vi "Tokenize.vi"(10 "Policy":T3=enum."lenient", 11 "Input":string="https://cdn-*.example.com/*.jpg") -> (0 "error out":errorcluster, 3 "Token List":T1[](array[typedef]))   [LabVIEW 2020, in "Stream.lvlib" / "URLPattern.lvclass"]
uses:
  URLPattern.lvclass
  Tokenize Policy.ctl
  Token.ctl
  Token Type.ctl
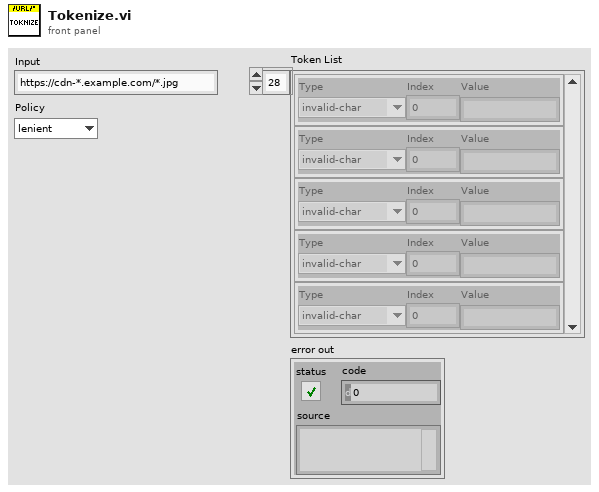
[diagram p1: front panel]
types:
  T1 = typedef "Stream.lvlib/URLPattern.lvclass/Token.ctl" = cluster{"Type":T2, "Index":i32, "Value":string}
  T2 = typedef "Stream.lvlib/URLPattern.lvclass/Token Type.ctl" = enum16{"invalid-char", "open", "close", "regexp", "name", "char", "escaped-char", "other-modifier", "asterisk", "end"}
  T3 = typedef "Stream.lvlib/URLPattern.lvclass/Tokenize Policy.ctl" = enum16{"strict", "lenient"}
  T4 = typedef "Stream.lvlib/URLPattern.lvclass/Tokenizer.ctl" = cluster{"Input":string, "Policy":T3, "Token List":refnum<queue>, "Index":i32, "Next Index":i32, "Code Point":u32, "Length":i32}
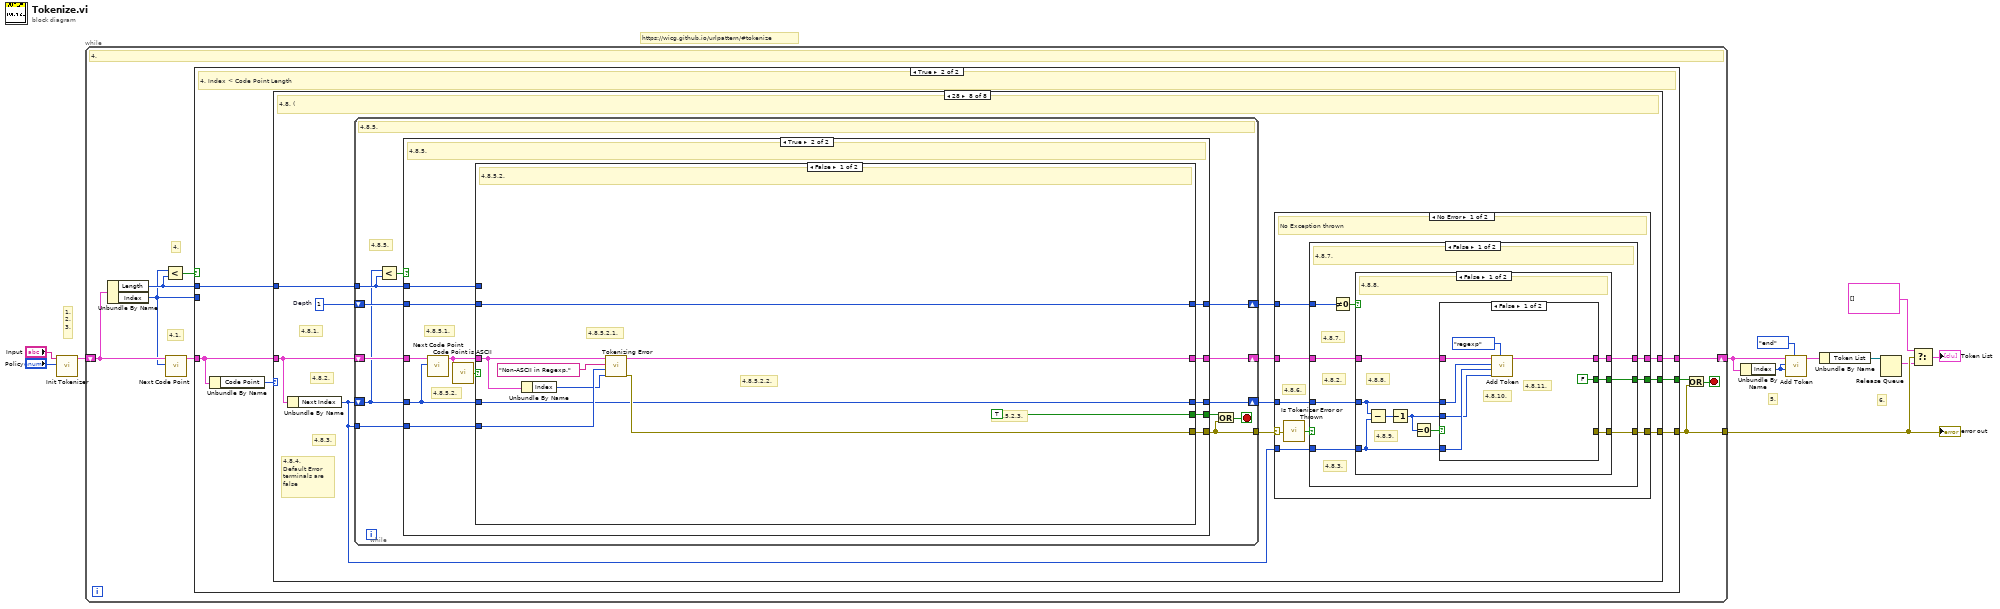
[diagram p0: block diagram]
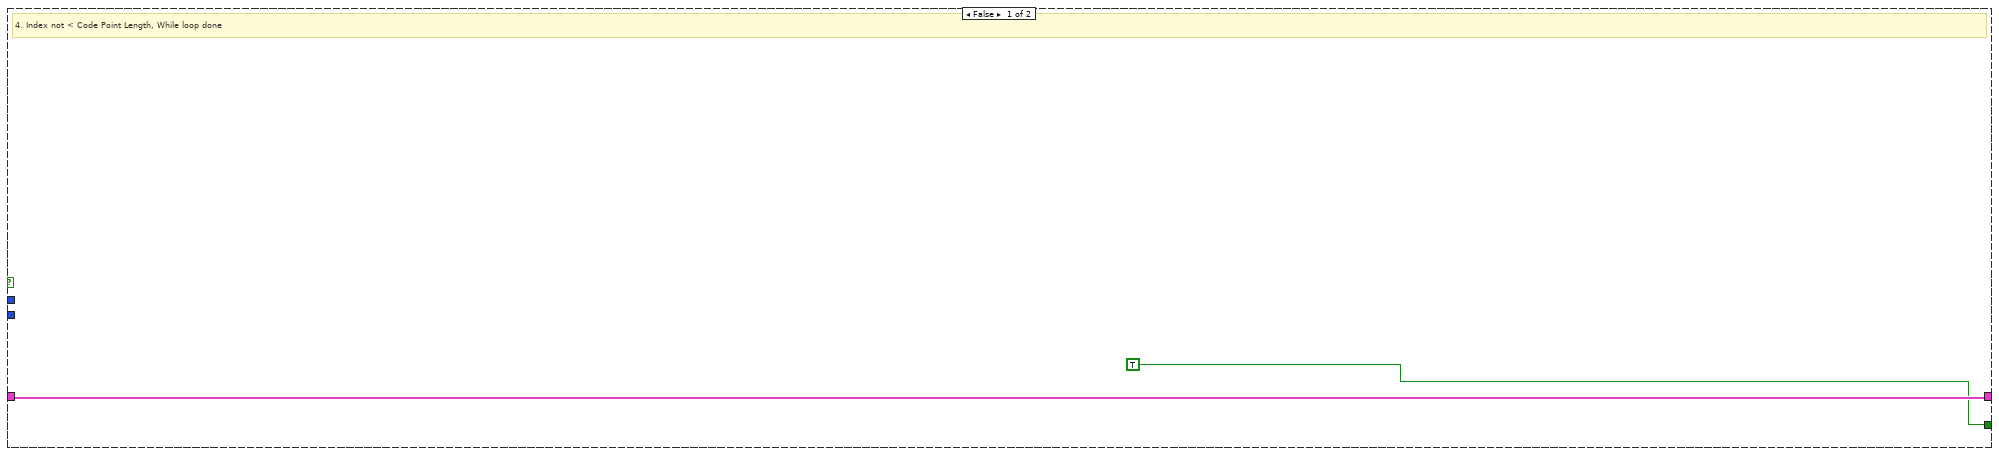
[diagram p2: hidden frame]
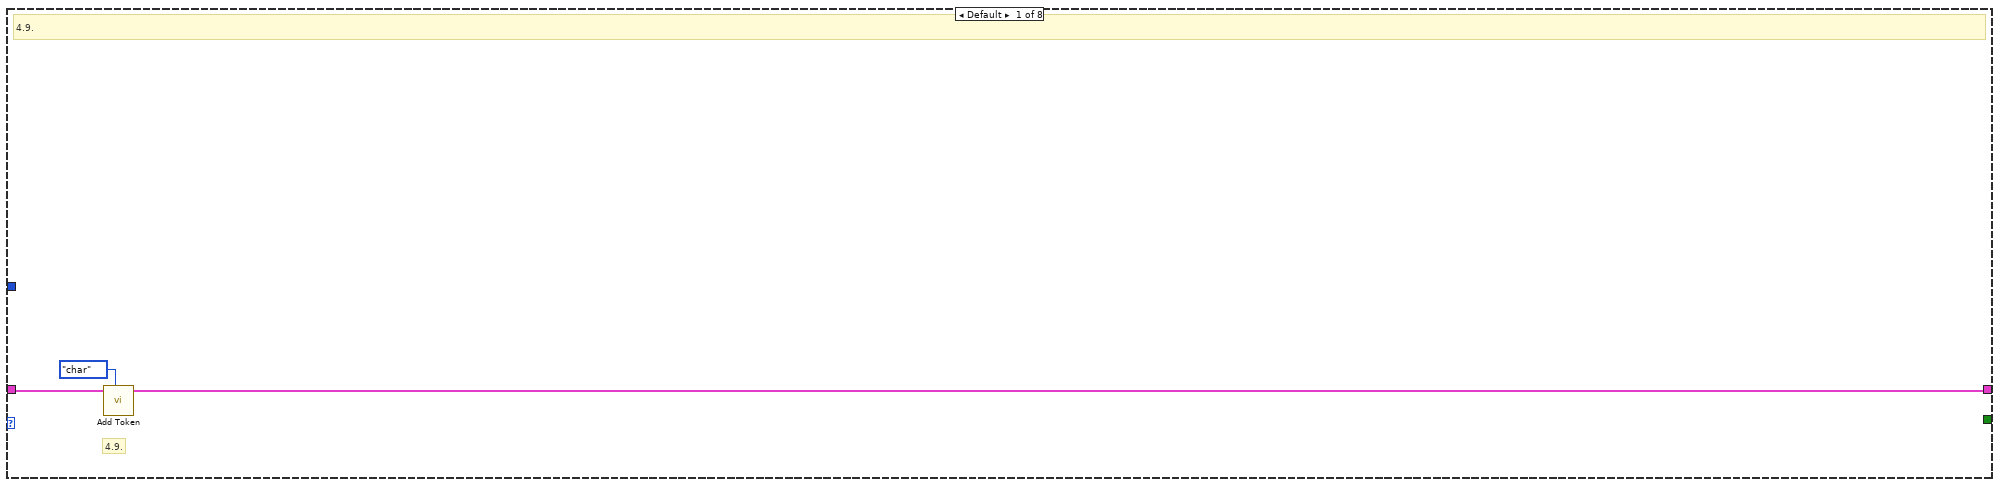
[diagram p3: hidden frame]
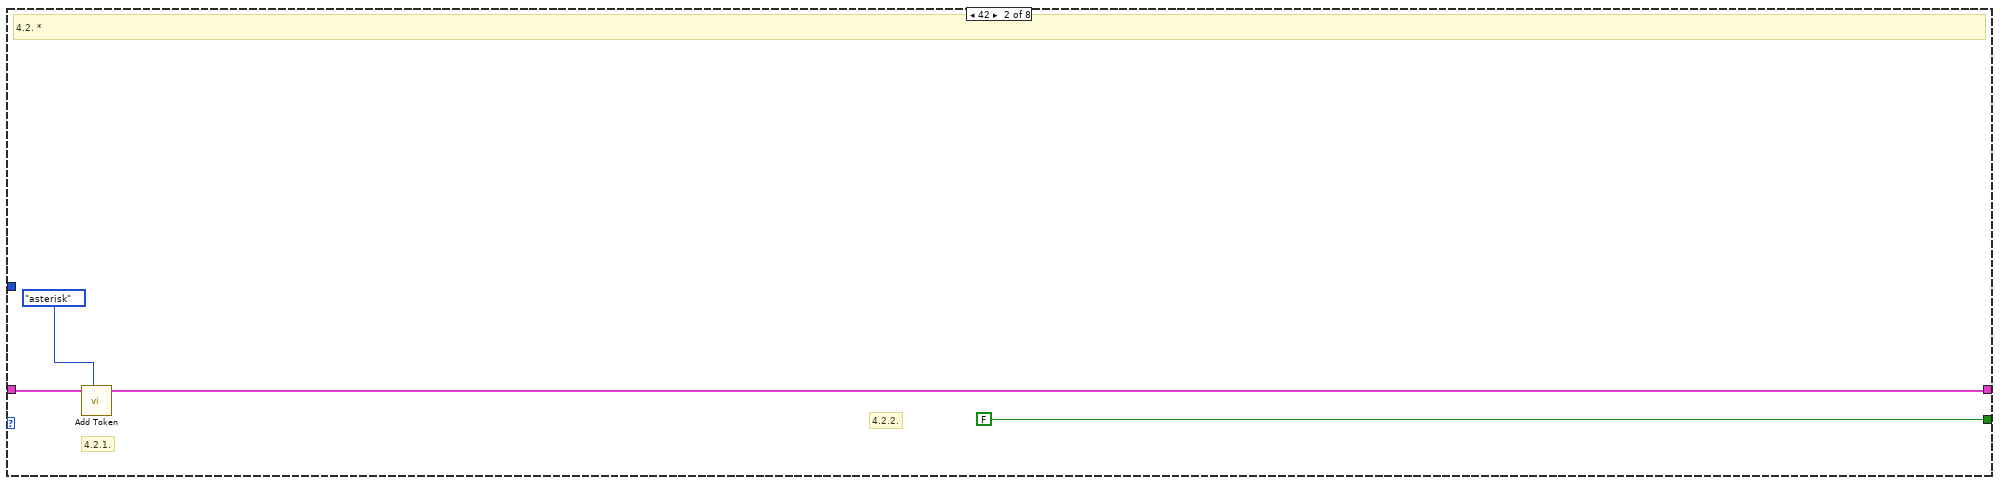
[diagram p4: hidden frame]
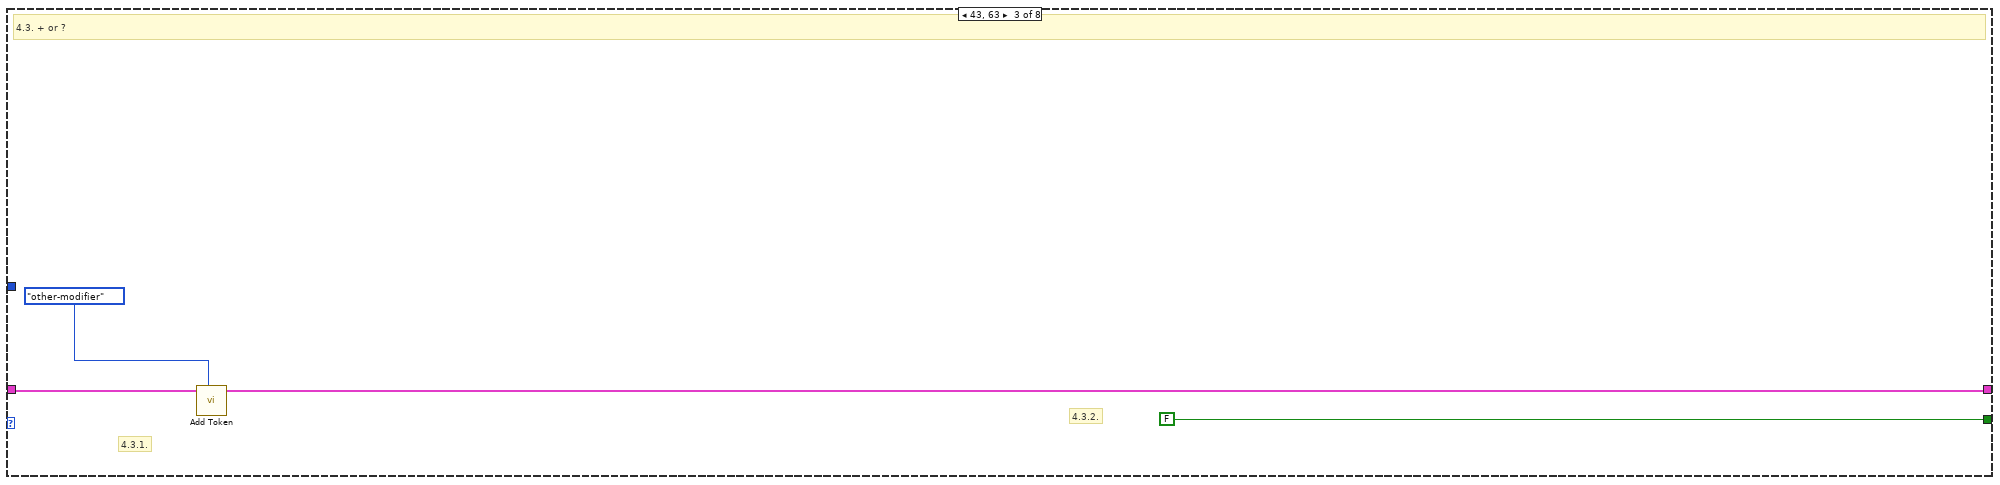
[diagram p5: hidden frame]
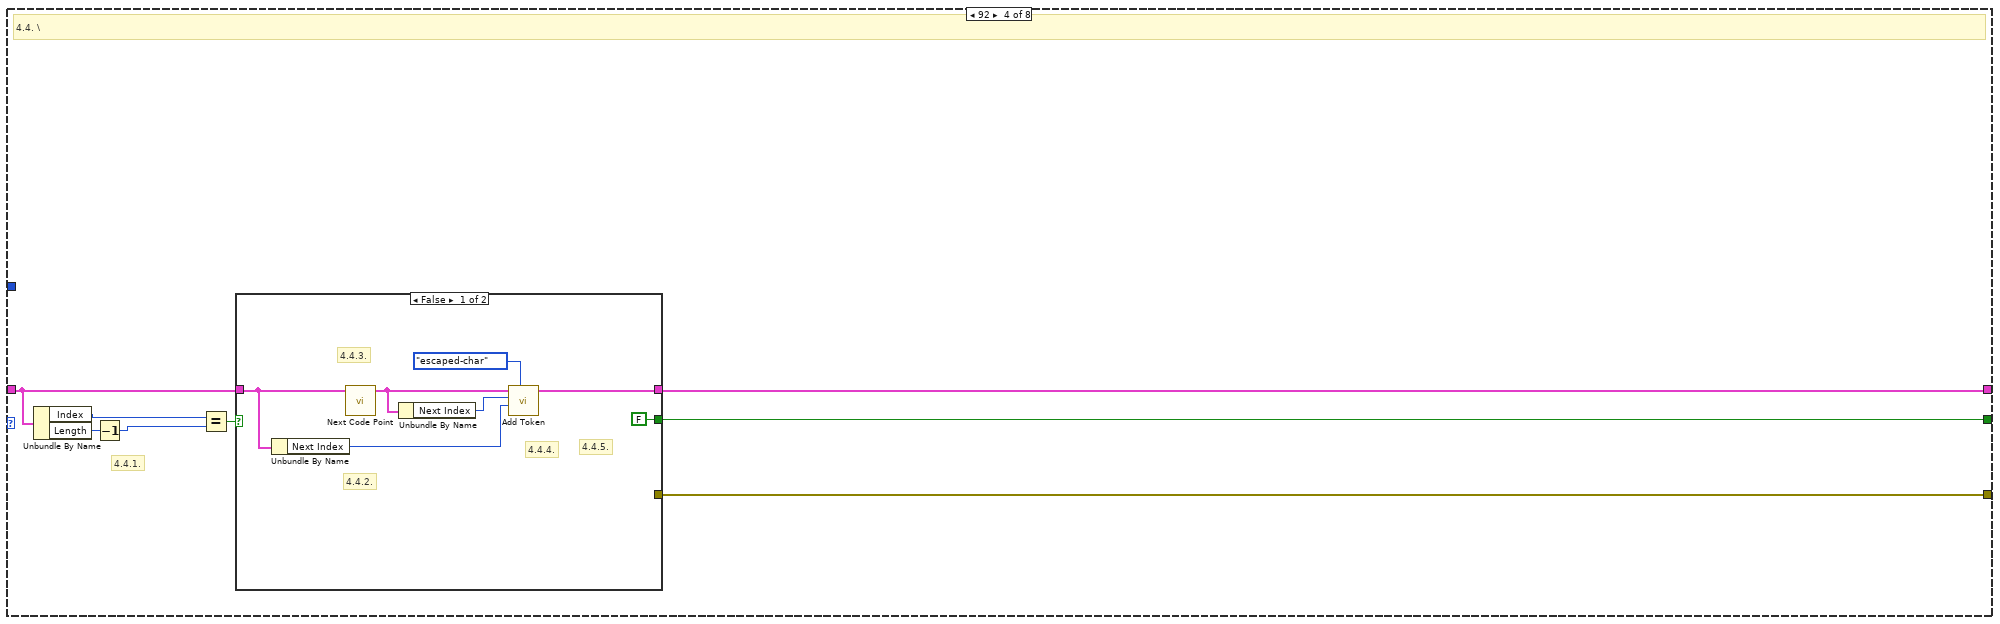
[diagram p6: hidden frame]
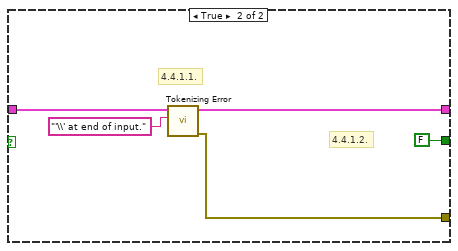
[diagram p7: hidden frame]
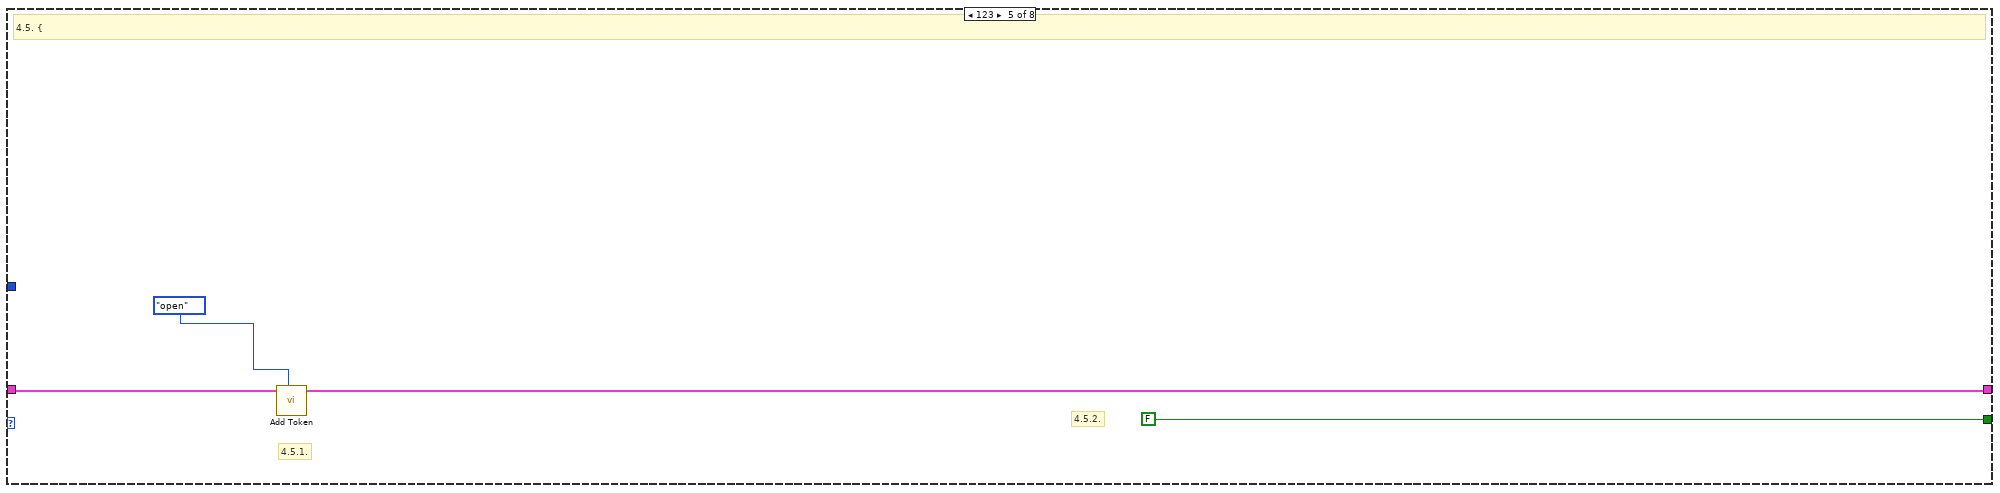
[diagram p8: hidden frame]
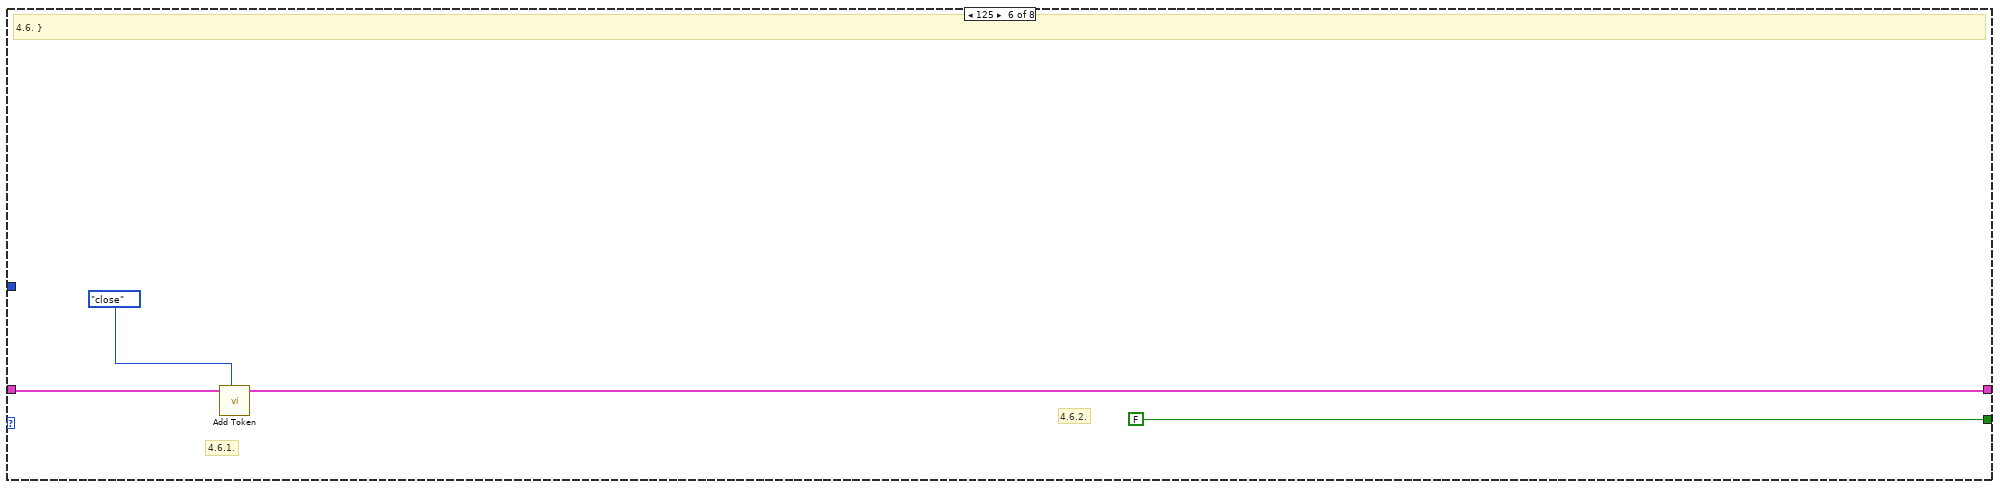
[diagram p9: hidden frame]
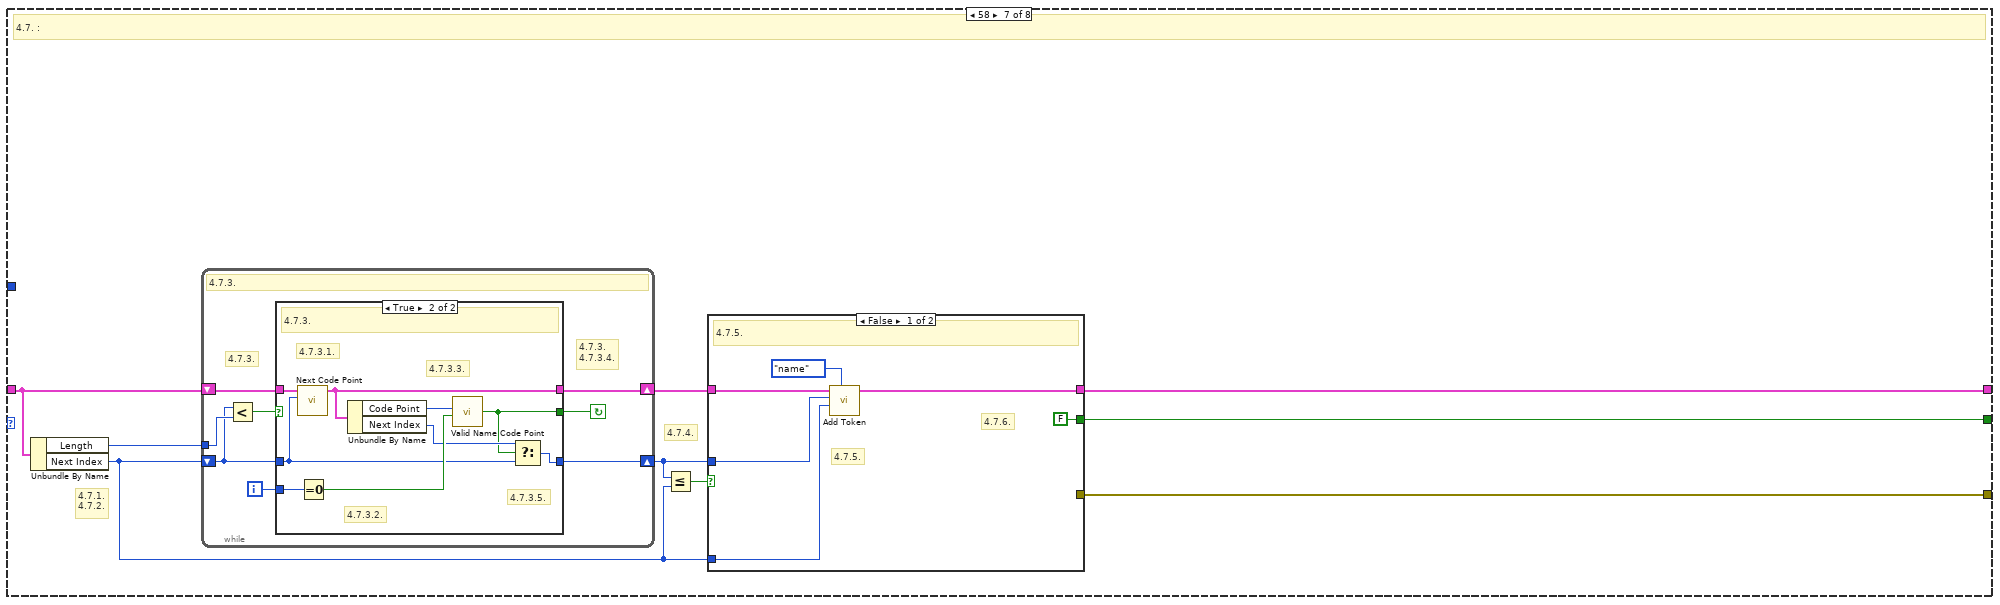
[diagram p10: hidden frame]
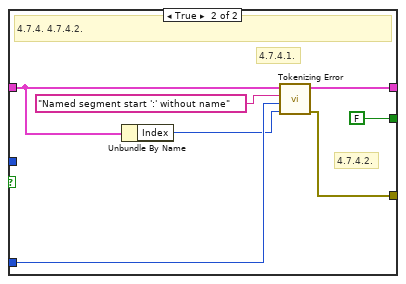
[diagram p11: hidden frame]
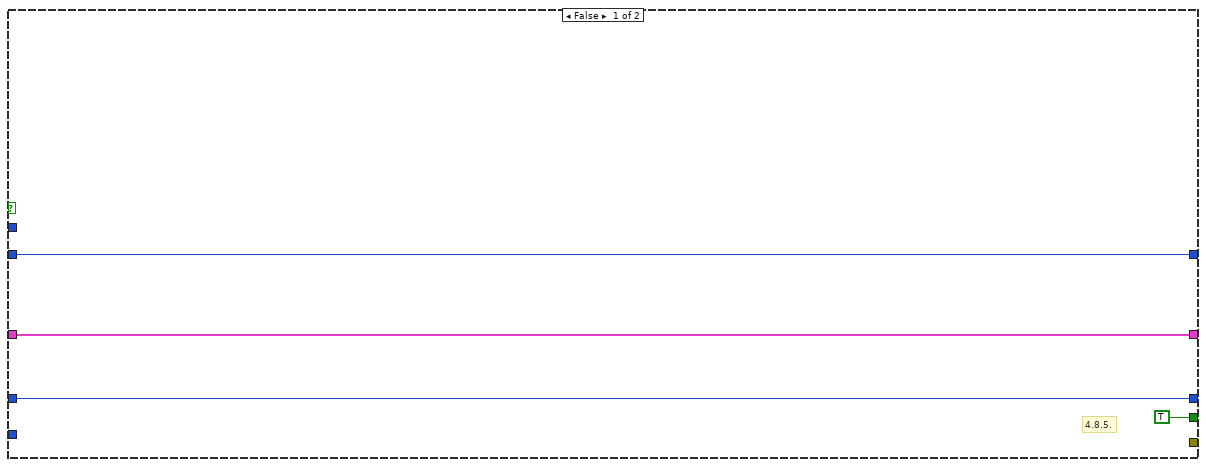
[diagram p13: hidden frame]
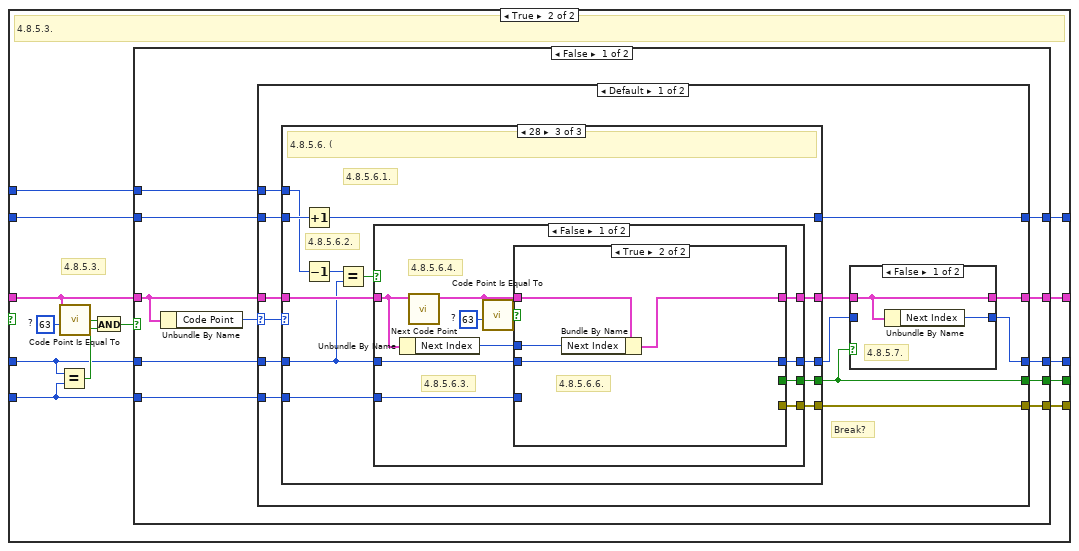
[diagram p14: hidden frame]
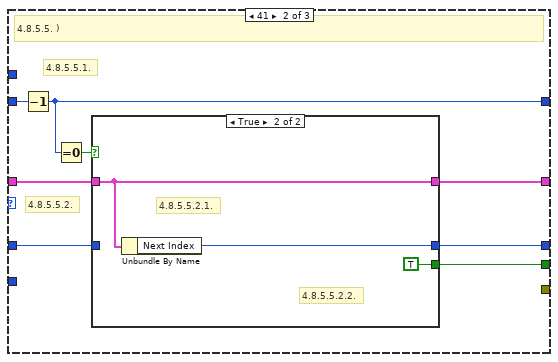
[diagram p17: hidden frame]
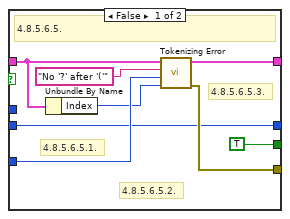
[diagram p19: hidden frame]
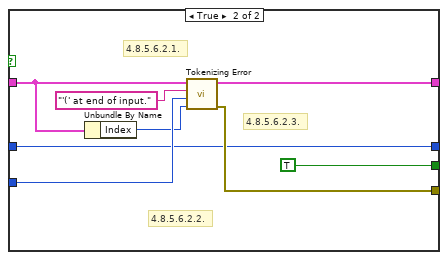
[diagram p20: hidden frame]
diagram:
  # "6."
  # "5."
  # "https://wicg.github.io/urlpattern/#tokenize"
  # "1.\n2.\n3."
  n1 = call "Init Tokenizer.vi"("Policy"="Policy", "Input"="Input") -> ("Tokenizer"=w9:T4)  [unwired: 9 in]
  n2 = while {
    shift-right: [w20] -> w2
    shift-left: w9 -> [w16]
    tunnel: [w17] -> w12
    stop <- w18 stop-if-true
    # "4.1."
    # "4."
    # "4."
    n3 = Unbundle By Name(w16) -> ("Length"=w14:i32, "Index"=w13:i32)
    n4 = Less?(x=w13, y=w14) -> (x < y?=w21:bool)
    n5 = call "Next Code Point.vi"("Index"=w13, "Tokenizer In"=w16) -> ("Tokenizer"=w15:T4)  [unwired: 9 in]
    n6 = case shown="True" w21 {
      tunnel: w13 -> [_ _]
      tunnel: w15 -> [w23 w28]
      tunnel: [w23 w27] -> w20
      tunnel: [TRUE w24] -> w19
      tunnel: [_ w26] -> w17
      tunnel: w14 -> [_ w25]
      frame False {
        # "4. Index not < Code Point Length, While loop done"
      }
      frame True {
        # "4. Index < Code Point Length"
        n7 = Unbundle By Name(w28) -> ("Code Point"=w29:u32)
        n8 = case shown="28" w29 {
          tunnel: w28 -> [w32 w36 w40 w45 w64 w68 w77 w120]
          tunnel: [w30 w34 w38 w42 w62 w66 w73 w114] -> w27
          tunnel: [_ _ _ w43 _ _ w72 w116] -> w26
          tunnel: w25 -> [_ _ _ _ _ _ _ w119]
          tunnel: [_ FALSE FALSE w41 FALSE FALSE w69 w117] -> w24
          frame Default {
            # "4.9."
            # "4.9."
            n9 = call "Add Token.vi"("Token Type"=Token_Type."char", "Tokenizer In"=w32) -> ("Tokenizer"=w30:T4)  [unwired: 9 in]
          }
          frame 42 {
            # "4.2.2."
            # "4.2.1."
            # "4.2. *"
            n10 = call "Add Token.vi"("Token Type"=Token_Type."asterisk", "Tokenizer In"=w36) -> ("Tokenizer"=w34:T4)  [unwired: 9 in]
          }
          frame 43, 63 {
            # "4.3.2."
            # "4.3.1."
            # "4.3. + or ?"
            n11 = call "Add Token.vi"("Token Type"=Token_Type."other-modifier", "Tokenizer In"=w40) -> ("Tokenizer"=w38:T4)  [unwired: 9 in]
          }
          frame 92 {
            # "4.4.1."
            # "4.4. \\"
            n12 = Unbundle By Name(w45) -> ("Index"=w46:i32, "Length"=w48:i32)
            n13 = Decrement(x=w48) -> (x-1=w47:i32)
            n14 = Equal?(x=w46, y=w47) -> (x = y?=w44:bool)
            n15 = case shown="False" w44 {
              tunnel: w45 -> [w55 w60]
              tunnel: [_ w57] -> w43
              tunnel: [w53 w58] -> w42
              tunnel: [FALSE FALSE] -> w41
              frame False {
                # "4.4.5."
                # "4.4.4."
                # "4.4.3."
                # "4.4.2."
                n16 = Unbundle By Name(w55) -> ("Next Index"=w52:i32)
                n17 = call "Next Code Point.vi"("Tokenizer In"=w55) -> ("Tokenizer"=w51:T4)  [unwired: 10 in]
                n18 = Unbundle By Name(w51) -> ("Next Index"=w50:i32)
                n19 = call "Add Token.vi"("Token Type"=Token_Type."escaped-char", "Value Position"=w52, "Next Position"=w50, "Tokenizer In"=w51) -> ("Tokenizer"=w53:T4)  [unwired: 7 in]
              }
              frame True {
                # "4.4.1.2."
                # "4.4.1.1."
                n20 = call "Tokenizing Error.vi"("Reason"="'\\' at end of input.", "Tokenizer In"=w60) -> ("error out"=w57:errorcluster, "Tokenizer"=w58:T4)  [unwired: 8 in]
              }
            }
          }
          frame 123 {
            # "4.5.2."
            # "4.5.1."
            # "4.5. {"
            n21 = call "Add Token.vi"("Token Type"=Token_Type."open", "Tokenizer In"=w64) -> ("Tokenizer"=w62:T4)  [unwired: 9 in]
          }
          frame 125 {
            # "4.6.2."
            # "4.6.1."
            # "4.6. }"
            n22 = call "Add Token.vi"("Token Type"=Token_Type."close", "Tokenizer In"=w68) -> ("Tokenizer"=w66:T4)  [unwired: 9 in]
          }
          frame 58 {
            # "4.7.4."
            # "4.7.1.\n4.7.2."
            # "4.7. :"
            n23 = Unbundle By Name(w77) -> ("Length"=w76:i32, "Next Index"=w71:i32)
            n24 = while {
              shift-right: [w95] -> w70
              shift-left: w71 -> [w92]
              shift-right: [w94] -> w74
              shift-left: w77 -> [w98]
              tunnel: w76 -> [w93]
              i -> [w97]
              stop <- w96 continue-if-true
              # "4.7.3.\n4.7.3.4."
              # "4.7.3."
              # "4.7.3."
              n25 = Less?(x=w92, y=w93) -> (x < y?=w91:bool)
              n26 = case shown="True" w91 {
                selector: w91 -> [w101 _]
                tunnel: w98 -> [w100 w110]
                tunnel: w97 -> [_ w109]
                tunnel: [w101 w105] -> w96
                tunnel: [w99 w104] -> w95
                tunnel: [w100 w103] -> w94
                tunnel: w92 -> [w99 w102]
                frame False {
                  # "4.7.3."
                }
                frame True {
                  # "4.7.3.5."
                  # "4.7.3.3."
                  # "4.7.3.2."
                  # "4.7.3.1."
                  # "4.7.3."
                  n27 = call "Next Code Point.vi"("Index"=w102, "Tokenizer In"=w110) -> ("Tokenizer"=w103:T4)  [unwired: 9 in]
                  n28 = Equal To 0?(x=w109) -> (x = 0?=w107:bool)
                  n29 = Unbundle By Name(w103) -> ("Code Point"=w108:u32, "Next Index"=w106:i32)
                  n30 = call "Valid Name Code Point.vi"("First"=w107, "Code Point"=w108) -> ("Valid?"=w105:bool)  [unwired: 2 in]
                  n31 = Select(t=w106, s=w105, f=w102) -> (s? t:f=w104:i32)
                }
              }
            }
            n32 = Less Or Equal?(x=w70, y=w71) -> (x <= y?=w75:bool)
            n33 = case shown="False" w75 {
              tunnel: w74 -> [w80 w86]
              tunnel: [w83 w90] -> w73
              tunnel: [_ w89] -> w72
              tunnel: w71 -> [w78 w87]
              tunnel: w70 -> [w81 _]
              tunnel: [FALSE FALSE] -> w69
              frame False {
                # "4.7.6."
                # "4.7.5."
                # "4.7.5."
                n34 = call "Add Token.vi"("Token Type"=Token_Type."name", "Value Position"=w78, "Next Position"=w81, "Tokenizer In"=w80) -> ("Tokenizer"=w83:T4)  [unwired: 7 in]
              }
              frame True {
                # "4.7.4.2."
                # "4.7.4.1."
                # "4.7.4. 4.7.4.2."
                n35 = Unbundle By Name(w86) -> ("Index"=w85:i32)
                n36 = call "Tokenizing Error.vi"("Value Position"=w85, "Next Position"=w87, "Reason"="Named segment start ':' without name", "Tokenizer In"=w86) -> ("error out"=w89:errorcluster, "Tokenizer"=w90:T4)  [unwired: 6 in]
              }
            }
          }
          frame 40 {
            w121 = 1  # Depth
            # "4.8.3."
            # "4.8.4.\nDefault Error terminals are false"
            # "4.8.1."
            # "4.8.2."
            # "4.8. ("
            n37 = Unbundle By Name(w120) -> ("Next Index"=w111:i32)
            n38 = while {
              shift-right: [w129] -> w112
              shift-left: w121 -> [w132]
              shift-right: [w128] -> w113
              shift-left: w111 -> [w126]
              tunnel: w111 -> [w131]
              shift-right: [w130] -> w115
              shift-left: w120 -> [w133]
              tunnel: [w122] -> w118
              tunnel: w119 -> [w127]
              stop <- w123 stop-if-true
              # "4.8.5."
              # "4.8.5."
              n39 = Less?(x=w126, y=w127) -> (x < y?=w125:bool)
              n40 = case shown="True" w125 {
                tunnel: w133 -> [w136 w149]
                tunnel: w132 -> [w137 w146]
                tunnel: w131 -> [_ w145]
                tunnel: [w136 w144] -> w130
                tunnel: [w137 w143] -> w129
                tunnel: [w135 w142] -> w128
                tunnel: [TRUE w141] -> w124
                tunnel: [_ w140] -> w122
                tunnel: w127 -> [_ w139]
                tunnel: w126 -> [w135 w138]
                frame False {
                  # "4.8.5."
                }
                frame True {
                  # "4.8.5.2."
                  # "4.8.5.1."
                  # "4.8.5."
                  n41 = call "Next Code Point.vi"("Index"=w138, "Tokenizer In"=w149) -> ("Tokenizer"=w147:T4)  [unwired: 9 in]
                  n42 = call "Code Point is ASCII.vi"("Tokenizer"=w147) -> ("ASCII?"=w148:bool)
                  n43 = case shown="False" w148 {
                    tunnel: w147 -> [w156 w168]
                    tunnel: w146 -> [w152 w162]
                    tunnel: w145 -> [w157 w166]
                    tunnel: [w154 w164] -> w140
                    tunnel: [w153 w165] -> w144
                    tunnel: [w152 w161] -> w143
                    tunnel: w138 -> [w151 w167]
                    tunnel: [w151 w163] -> w142
                    tunnel: w139 -> [_ w160]
                    tunnel: [TRUE w159] -> w141
                    frame False {
                      # "4.8.5.2.3."
                      # "4.8.5.2.2."
                      # "4.8.5.2.1."
                      # "4.8.5.2."
                      n44 = Unbundle By Name(w156) -> ("Index"=w155:i32)
                      n45 = call "Tokenizing Error.vi"("Value Position"=w155, "Next Position"=w157, "Reason"="Non-ASCII in Regexp.", "Tokenizer In"=w156) -> ("error out"=w154:errorcluster, "Tokenizer"=w153:T4)  [unwired: 6 in]
                    }
                    frame True {
                      w172 = u32 63  # ?
                      # "4.8.5.3."
                      # "4.8.5.3."
                      n46 = Equal?(x=w167, y=w166) -> (x = y?=w170:bool)
                      n47 = call "Code Point Is Equal To.vi"("Code Point"=w172, "Tokenizer"=w168) -> ("Code Point Equals?"=w171:bool)  [unwired: 2 in]
                      n48 = And(x=w171, y=w170) -> (x .and. y?=w169:bool)
                      n49 = case shown="False" w169 {
                        tunnel: w168 -> [w175 w311]
                        tunnel: w167 -> [w182 w307]
                        tunnel: w166 -> [w179 w312]
                        tunnel: [w177 w309] -> w165
                        tunnel: [w178 w308] -> w164
                        tunnel: [w176 w307] -> w163
                        tunnel: w162 -> [w183 w306]
                        tunnel: [w180 w306] -> w161
                        tunnel: w160 -> [w181 _]
                        tunnel: [w173 TRUE] -> w159
                        frame False {
                          n50 = Unbundle By Name(w175) -> ("Code Point"=w174:u32)
                          n51 = case shown="Default" w174 {
                            selector: w174 -> [w196 _]
                            tunnel: w175 -> [w191 w267]
                            tunnel: w183 -> [w194 w268]
                            tunnel: w182 -> [w193 w263]
                            tunnel: w181 -> [w195 w271]
                            tunnel: [w190 w261] -> w180
                            tunnel: w179 -> [w192 w266]
                            tunnel: [w189 w265] -> w178
                            tunnel: [w185 w264] -> w177
                            tunnel: [w184 w262] -> w176
                            tunnel: [w186 w260] -> w173
                            frame Default {
                              # "Break?"
                              n52 = case shown="28" w196 {
                                tunnel: w195 -> [_ _ w226]
                                tunnel: w194 -> [w202 w211 w228]
                                tunnel: w193 -> [w201 w204 w218]
                                tunnel: w192 -> [_ _ w221]
                                tunnel: w191 -> [w203 w208 w224]
                                tunnel: [w203 w205 w222] -> w188
                                tunnel: [w202 w210 w227] -> w190
                                tunnel: [w201 w207 w217] -> w187
                                tunnel: [_ w206 w219] -> w186
                                tunnel: [_ _ w220] -> w189
                                frame Default {
                                }
                                frame 41 {
                                # "4.8.5.5.2."
                                # "4.8.5.5.1."
                                # "4.8.5.5. )"
                                n53 = Decrement(x=w211) -> (x-1=w210:i32)
                                n54 = Equal To 0?(x=w210) -> (x = 0?=w209:bool)
                                n55 = case shown="True" w209 {
                                tunnel: w208 -> [w213 w214]
                                tunnel: [w212 w216] -> w207
                                tunnel: [_ TRUE] -> w206
                                tunnel: [w213 w214] -> w205
                                tunnel: w204 -> [w212 _]
                                frame False {
                                }
                                frame True {
                                # "4.8.5.5.2.2."
                                # "4.8.5.5.2.1."
                                n56 = Unbundle By Name(w214) -> ("Next Index"=w216:i32)
                                }
                                }
                                }
                                frame 40 {
                                # "4.8.5.6.2."
                                # "4.8.5.6.1."
                                # "4.8.5.6. ("
                                n57 = Increment(x=w228) -> (x+1=w227:i32)
                                n58 = Decrement(x=w226) -> (x-1=w225:i32)
                                n59 = Equal?(x=w225, y=w218) -> (x = y?=w223:bool)
                                n60 = case shown="False" w223 {
                                tunnel: w224 -> [w239 w256]
                                tunnel: [w232 w259] -> w222
                                tunnel: w221 -> [w231 w257]
                                tunnel: [w233 w254] -> w220
                                tunnel: [w230 TRUE] -> w219
                                tunnel: w218 -> [w236 w252]
                                tunnel: [w229 w252] -> w217
                                frame False {
                                w238 = u32 63  # ?
                                # "4.8.5.6.4."
                                # "4.8.5.6.3."
                                n61 = Unbundle By Name(w239) -> ("Next Index"=w235:i32)
                                n62 = call "Next Code Point.vi"("Tokenizer In"=w239) -> ("Tokenizer"=w234:T4)  [unwired: 10 in]
                                n63 = call "Code Point Is Equal To.vi"("Code Point"=w238, "Tokenizer"=w234) -> ("Code Point Equals?"=w237:bool)  [unwired: 2 in]
                                n64 = case shown="True" w237 {
                                tunnel: w236 -> [w240 w248]
                                tunnel: w235 -> [_ w250]
                                tunnel: w234 -> [w243 w251]
                                tunnel: [w247 _] -> w233
                                tunnel: [w246 w249] -> w232
                                tunnel: w231 -> [w244 _]
                                tunnel: [TRUE _] -> w230
                                tunnel: [w240 w248] -> w229
                                frame False {
                                # "4.8.5.6.5.3."
                                # "4.8.5.6.5.2."
                                # "4.8.5.6.5.1."
                                # "4.8.5.6.5."
                                n65 = Unbundle By Name(w243) -> ("Index"=w242:i32)
                                n66 = call "Tokenizing Error.vi"("Value Position"=w242, "Next Position"=w244, "Reason"="No '?' after '('", "Tokenizer In"=w243) -> ("error out"=w247:errorcluster, "Tokenizer"=w246:T4)  [unwired: 6 in]
                                }
                                frame True {
                                # "4.8.5.6.6."
                                n67 = Bundle By Name(cluster=w251, "Next Index"=w250) -> (w249:T4)
                                }
                                }
                                }
                                frame True {
                                # "4.8.5.6.2.3."
                                # "4.8.5.6.2.2."
                                # "4.8.5.6.2.1."
                                n68 = Unbundle By Name(w256) -> ("Index"=w255:i32)
                                n69 = call "Tokenizing Error.vi"("Value Position"=w255, "Next Position"=w257, "Reason"="'(' at end of input.", "Tokenizer In"=w256) -> ("error out"=w254:errorcluster, "Tokenizer"=w259:T4)  [unwired: 6 in]
                                }
                                }
                                }
                              }
                              n70 = case shown="False" w186 {
                                tunnel: w188 -> [w197 w200]
                                tunnel: w187 -> [_ w199]
                                tunnel: [w197 w200] -> w185
                                tunnel: [w198 w199] -> w184
                                frame False {
                                # "4.8.5.7."
                                n71 = Unbundle By Name(w197) -> ("Next Index"=w198:i32)
                                }
                                frame True {
                                }
                              }
                            }
                            frame 92 {
                              # "4.8.5.4.1."
                              # "4.8.5.4. \\"
                              n72 = Decrement(x=w271) -> (x-1=w270:i32)
                              n73 = Equal?(x=w270, y=w263) -> (x = y?=w269:bool)
                              n74 = case shown="False" w269 {
                                tunnel: w268 -> [w279 w297]
                                tunnel: w267 -> [w282 w302]
                                tunnel: w266 -> [w274 w303]
                                tunnel: [w275 w300] -> w265
                                tunnel: [w277 w299] -> w264
                                tunnel: w263 -> [w278 w298]
                                tunnel: [w273 w298] -> w262
                                tunnel: [w276 w297] -> w261
                                tunnel: [w272 TRUE] -> w260
                                frame False {
                                # "4.8.5.4.2."
                                n75 = call "Next Code Point.vi"("Tokenizer In"=w282) -> ("Tokenizer"=w280:T4)  [unwired: 10 in]
                                n76 = call "Code Point is ASCII.vi"("Tokenizer"=w280) -> ("ASCII?"=w281:bool)
                                n77 = case shown="True" w281 {
                                tunnel: w280 -> [w286 w293]
                                tunnel: w279 -> [w289 w294]
                                tunnel: w278 -> [w284 _]
                                tunnel: [w290 w293] -> w277
                                tunnel: [w289 w294] -> w276
                                tunnel: [w288 _] -> w275
                                tunnel: w274 -> [w287 _]
                                tunnel: [w284 w295] -> w273
                                tunnel: [TRUE FALSE] -> w272
                                frame False {
                                # "4.8.5.4.3.3."
                                # "4.8.5.4.3.2."
                                # "4.8.5.4.3.1."
                                # "4.8.5.4.3."
                                n78 = Unbundle By Name(w286) -> ("Index"=w285:i32)
                                n79 = call "Tokenizing Error.vi"("Value Position"=w285, "Next Position"=w287, "Reason"="Invalid escape in Regexp.", "Tokenizer In"=w286) -> ("error out"=w288:errorcluster, "Tokenizer"=w290:T4)  [unwired: 6 in]
                                }
                                frame True {
                                # "4.8.5.4.5."
                                # "4.8.5.4.4."
                                # "4.8.5.4.4."
                                n80 = Unbundle By Name(w293) -> ("Next Index"=w295:i32)
                                }
                                }
                                }
                                frame True {
                                # "4.8.5.4.1.3."
                                # "4.8.5.4.1.2."
                                # "4.8.5.4.1.1."
                                n81 = Unbundle By Name(w302) -> ("Index"=w301:i32)
                                n82 = call "Tokenizing Error.vi"("Value Position"=w301, "Next Position"=w303, "Reason"="Invalid '\\' at end of Regexp input", "Tokenizer In"=w302) -> ("error out"=w300:errorcluster, "Tokenizer"=w299:T4)  [unwired: 6 in]
                                }
                              }
                            }
                          }
                        }
                        frame True {
                          # "4.8.5.3.3."
                          # "4.8.5.3.2."
                          # "4.8.5.3.1."
                          # "4.8.5.3."
                          n83 = Unbundle By Name(w311) -> ("Index"=w310:i32)
                          n84 = call "Tokenizing Error.vi"("Value Position"=w310, "Next Position"=w312, "Reason"="'\\?' invalid in Regexp", "Tokenizer In"=w311) -> ("error out"=w308:errorcluster, "Tokenizer"=w309:T4)  [unwired: 6 in]
                        }
                      }
                    }
                  }
                }
              }
              n85 = Or(x=w124, y=w122) -> (x .or. y?=w123:bool)
            }
            n86 = case shown="No Error" w118 {
              selector: w118 -> [w315 w364]
              tunnel: [w317 _] -> w117
              tunnel: [w319 w364] -> w116
              tunnel: w115 -> [w321 w363]
              tunnel: [w318 w363] -> w114
              tunnel: w113 -> [w316 _]
              tunnel: w112 -> [w322 _]
              tunnel: w111 -> [w320 _]
              frame No Error {
                # "4.8.6."
                # "No Exception thrown"
                n87 = call "Is Tokenizer Error or Thrown.vi"("Error"=w315) -> ("Tokenizer Error?"=w314:bool)  [unwired: 1 out]
                n88 = case shown="False" w314 {
                  tunnel: w322 -> [w330 _]
                  tunnel: w321 -> [w328 w361]
                  tunnel: w320 -> [w327 _]
                  tunnel: [w326 _] -> w319
                  tunnel: [w325 w361] -> w318
                  tunnel: [w324 FALSE] -> w317
                  tunnel: w316 -> [w323 _]
                  frame False {
                    # "4.8.2."
                    # "4.8.3."
                    # "4.8.7."
                    # "4.8.7."
                    n89 = Not Equal To 0?(x=w330) -> (x != 0?=w329:bool)
                    n90 = case shown="False" w329 {
                      tunnel: w328 -> [w336 w359]
                      tunnel: w327 -> [w332 w357]
                      tunnel: [w334 w356] -> w326
                      tunnel: [w335 w355] -> w325
                      tunnel: [w333 FALSE] -> w324
                      tunnel: w323 -> [w331 _]
                      frame False {
                        # "4.8.9."
                        # "4.8.8."
                        # "4.8.8."
                        n91 = Subtract(x=w331, y=w332) -> (x-y=w339:i32)
                        n92 = Decrement(x=w339) -> (x-1=w337:i32)
                        n93 = Equal To 0?(x=w337) -> (x = 0?=w338:bool)
                        n94 = case shown="False" w338 {
                          tunnel: w337 -> [w342 _]
                          tunnel: w336 -> [w346 w349]
                          tunnel: [w341 w353] -> w335
                          tunnel: [_ w352] -> w334
                          tunnel: [FALSE FALSE] -> w333
                          tunnel: w332 -> [w343 w347]
                          tunnel: w331 -> [w344 _]
                          frame False {
                            # "4.8.11."
                            # "4.8.10."
                            n95 = call "Add Token.vi"("Token Type"=Token_Type."regexp", "Length"=w342, "Value Position"=w343, "Next Position"=w344, "Tokenizer In"=w346) -> ("Tokenizer"=w341:T4)  [unwired: 6 in]
                          }
                          frame True {
                            # "4.8.9.2."
                            # "4.8.9.1."
                            # "4.8.9."
                            n96 = Unbundle By Name(w349) -> ("Index"=w348:i32)
                            n97 = call "Tokenizing Error.vi"("Value Position"=w348, "Next Position"=w347, "Reason"="Empty Regexp", "Tokenizer In"=w349) -> ("error out"=w352:errorcluster, "Tokenizer"=w353:T4)  [unwired: 6 in]
                          }
                        }
                      }
                      frame True {
                        # "4.8.7.2."
                        # "4.8.7.1."
                        # "4.8.7."
                        n98 = Unbundle By Name(w359) -> ("Index"=w358:i32)
                        n99 = call "Tokenizing Error.vi"("Value Position"=w358, "Next Position"=w357, "Reason"="Unfinished Regexp", "Tokenizer In"=w359) -> ("error out"=w356:errorcluster, "Tokenizer"=w355:T4)  [unwired: 6 in]
                      }
                    }
                  }
                  frame True {
                    # "4.8.6."
                    # "4.8.6."
                  }
                }
              }
              frame Error {
                # "Exception thrown"
                # "Exception thrown"
              }
            }
          }
        }
      }
    }
    n100 = Or(x=w19, y=w17) -> (x .or. y?=w18:bool)
  }
  "error out" <- w12
  n101 = Unbundle By Name(w2) -> ("Index"=w1:i32)
  n102 = call "Add Token.vi"("Token Type"=Token_Type."end", "Value Position"=w1, "Next Position"=w1, "Tokenizer In"=w2) -> ("Tokenizer"=w4:T4)  [unwired: 7 in]
  n103 = Unbundle By Name(w4) -> ("Token List"=w8:refnum<queue>)
  n104 = Release Queue(queue=w8) -> (remaining elements=w7:T1[])  [unwired: 2 in, 2 out]
  n105 = Select(t=T1[] [], s=w12, f=w7) -> (s? t:f=→"Token List":T1[])
